vi "Actor Core.vi"(8 "error in":errorcluster, 11 "State in":refnum<class "Door Controller.lvclass">) -> (0 "error out":errorcluster, 3 "Actor out":refnum<class "Actor.lvclass">)   [LabVIEW 2020, in "Door Controller.lvlib" / "Door Controller.lvclass"]
doc: "(<B>Filename</B>: Actor Framework.lvlib:Actor.lvclass:Actor Core.vi)\n\nThis override invokes Entry.vi on the initial state, prior to calling the parent Actor Core. Adding this behavior to Actor Core (instead of an override of Pre Launch Init.vi) allows the initial state to launch a nested actor as part of its entry behavior.\n\nReceives messages to the actor, reacts to them, and initiates any error handling that may shut the actor down.\n\nDescendant classes may override this VI to append parallel tasks for the actor to complete while it handles messages. Overrides use the Call Parent Method node."
uses:
  Door Controller.lvclass
  C:/Program Files/National Instruments/LabVIEW 2020/vi.lib/ActorFramework/Actor/Actor.lvclass
  <vilib>/ActorFramework/Actor/Actor.lvclass
  Door Hardware/Door Hardware/Door Hardware.lvclass
  Door Controller.lvclass/Door Controller.ctl
  Application/Application/Application.lvclass
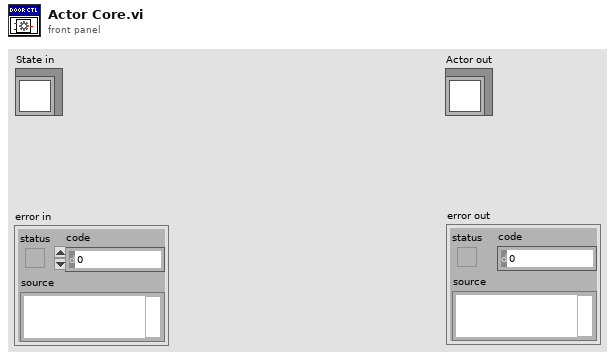
[diagram p1: front panel]
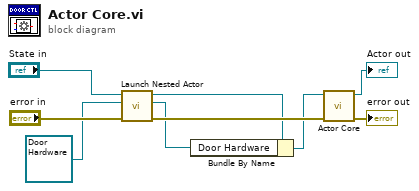
[diagram p0: block diagram]
diagram:
  n1 = call <vilib>:"Launch Nested Actor.vi"("error in (no error)"="error in", "Nested Actor"=refnum<class "Door Hardware.lvclass"> refnum ("Door Hardware.lvlib:Door Hardware.lvclass"), "Caller Actor in"="State in") -> ("error out"=w6:errorcluster, "Nested Actor's Enqueuer"=w1:refnum<class "Message Enqueuer.lvclass">, "Caller Actor out"=w3:refnum<class "Door Controller.lvclass">)  [unwired: 6 in]
  n2 = Bundle By Name(cluster=w3, "Door Hardware"=w1) -> (w2:refnum<class "Door Controller.lvclass">)
  n3 = call-parent "Actor Core.vi"("error in"=w6, "Actor in"=w2) -> ("error out"=→"error out":errorcluster, "Actor out"=→"Actor out":refnum<class "Actor.lvclass">)  [unwired: 8 in]
